vi "cmdmain.vi"(10 "EXE Name":string, 11 "command line arguments":T1) -> (0 "error out":errorcluster)   [LabVIEW 2018]
uses:
  arguments.ctl
  <vilib>/Utility/sysdir.llb/Get System Directory.vi
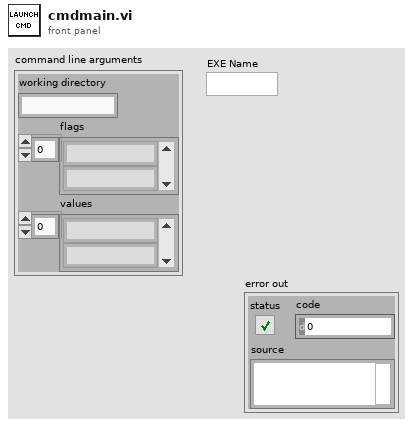
[diagram p1: front panel]
types:
  T1 = typedef "arguments.ctl" = cluster{"working directory":string, "flags":string[], "values":string[]}
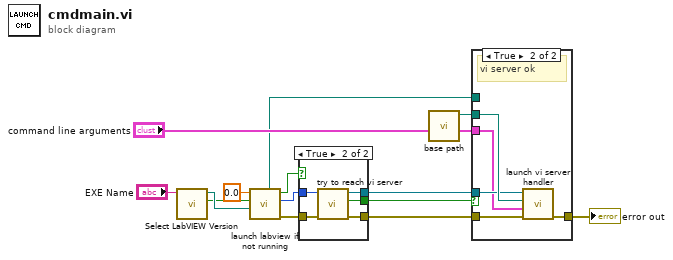
[diagram p0: block diagram]
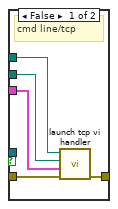
[diagram p2: hidden frame]
diagram:
  n1 = call "Select LabVIEW Version.vi"("EXE Name"="EXE Name") -> ("Exe Path Specified"=w4:bool, "LabVIEW Path"=w5:path)  [unwired: 9 in]
  n2 = call "launch labview if not running.vi"("exe path"=w5, "lv path specified"=w4, "desired lv version"=0.0) -> ("error out"=w13:errorcluster, "port"=w12:u32, "vi server available"=w14:bool, "labview directory"=w1:path)  [unwired: 4 in, 1 out]
  n3 = case shown="True" w14 {
    selector: w14 -> [w15 _]
    tunnel: w13 -> [w16 w20]
    tunnel: w12 -> [_ w21]
    tunnel: [w16 w17] -> w9
    tunnel: [w15 w18] -> w11
    tunnel: [_ w19] -> w10
    frame False {
    }
    frame True {
      n4 = call "try to reach vi server.vi"("error in"=w20, "port"=w21) -> ("error out"=w17:errorcluster, "connected"=w18:bool, "Application out"=w19:refnum<vi>)  [unwired: 7 in]
    }
  }
  n5 = call "base path.vi"() -> ("base path"=w7:path)  [unwired: 11 in]
  n6 = case shown="True" w11 {
    tunnel: w10 -> [_ w29]
    tunnel: w7 -> [w26 w31]
    tunnel: w9 -> [w22 w30]
    tunnel: "command line arguments" -> [w25 w28]
    tunnel: [w24 w27] -> w8
    tunnel: w1 -> [w23 _]
    frame False {
      # "cmd line/tcp"
      n7 = call "launch tcp vi handler.vi"("error in"=w22, "command line arguments"=w25, "base path"=w26, "labview directory"=w23) -> ("error out"=w24:errorcluster)  [unwired: 7 in]
    }
    frame True {
      # "vi server ok"
      n8 = call "launch vi server handler.vi"("error in"=w30, "command line arguments"=w28, "base path"=w31, "Application in"=w29) -> ("error out"=w27:errorcluster)  [unwired: 7 in]
    }
  }
  "error out" <- w8
